vi "Looper.vi"(8 "error in (no error)":errorcluster, 11 "RSA in":refnum<class "RSA.lvclass">) -> (0 "error out":errorcluster, 3 "RSA out":refnum<class "RSA.lvclass">)   [LabVIEW 2012, in "RSA.lvclass"]
uses:
  RSA.lvclass
  <vilib>/Distrio/Murmex/GenericMessage/GenericMessage.lvclass
  <vilib>/Distrio/Murmex/Murmex/Murmex.lvclass
  <vilib>/Distrio/Murmex/ResetMessage/ResetMessage.lvclass
  <vilib>/Distrio/Murmex/StopMessage/StopMessage.lvclass
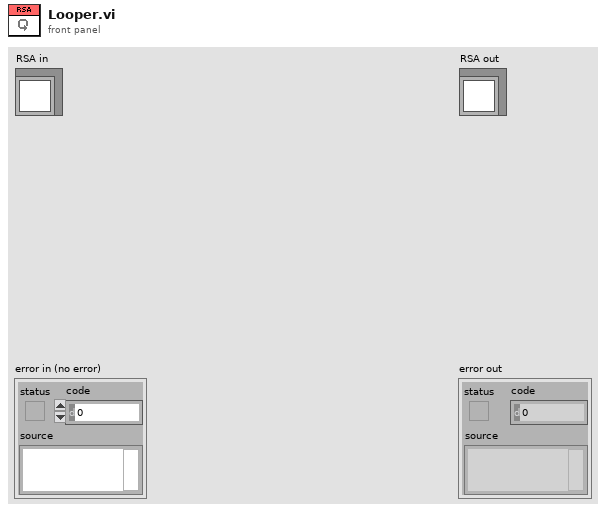
[diagram p1: front panel]
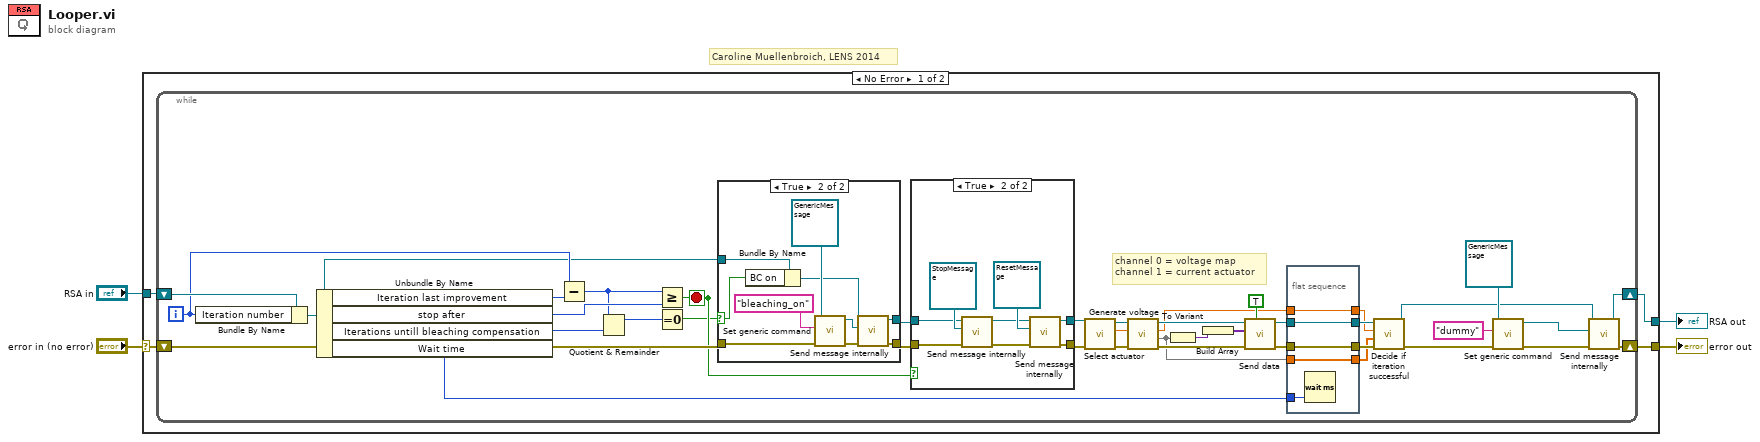
[diagram p0: block diagram]
diagram:
  # "Caroline Muellenbroich, LENS 2014"
  n1 = case shown="No Error" "error in (no error)" {
    selector: "error in (no error)" -> [w7 w77]
    tunnel: [w5 w77] -> w3
    tunnel: [w6 w76] -> w1
    tunnel: "RSA in" -> [w8 w76]
    frame No Error {
      n2 = while {
        shift-right: [w16] -> w6
        shift-left: w8 -> [w48]
        shift-right: [w15] -> w5
        shift-left: w7 -> [w44]
        i -> [w47]
        stop <- w40 stop-if-true
        # "channel 0 = voltage map\nchannel 1 = current actuator"
        n3 = Bundle By Name(cluster=w48, "Iteration number"=w47) -> (w45:refnum<class "RSA.lvclass">)
        n4 = Unbundle By Name(w45) -> ("Iteration last improvement"=w41:i32, "stop after"=w46:i32, "Iterations untill bleaching compensation"=w25:i32, "Wait time"=w27:u32)
        n5 = Subtract(x=w47, y=w41) -> (x-y=w26:i32)
        n6 = Quotient & Remainder(x=w26, y=w25) -> (x-y*floor(x/y)=w24:i32)  [unwired: 1 out]
        n7 = Greater Or Equal?(x=w26, y=w46) -> (x >= y?=w40:bool)
        n8 = Equal To 0?(x=w24) -> (x = 0?=w18:bool)
        n9 = case shown="True" w18 {
          selector: w18 -> [_ w56]
          tunnel: w45 -> [w55 w59]
          tunnel: [w55 w61] -> w42
          tunnel: w44 -> [w54 w62]
          tunnel: [w54 w60] -> w43
          frame False {
          }
          frame True {
            n10 = Bundle By Name(cluster=w59, "BC on"=w56) -> (w58:refnum<class "RSA.lvclass">)
            n11 = call <vilib>:"Set generic command.vi"("error in (no error)"=w62, "generic command"="bleaching_on", "GenericMessage in"=refnum<class "GenericMessage.lvclass"> refnum ("Murmex.lvlib:GenericMessage")) -> ("error out"=w64:errorcluster, "GenericMessage out"=w57:refnum<class "GenericMessage.lvclass">)  [unwired: 7 in]
            n12 = call <vilib>:"Send message internally.vi"("error in (no error)"=w64, "Message"=w57, "Murmex in"=w58) -> ("error out"=w60:errorcluster, "Murmex out"=w61:refnum<class "RSA.lvclass">)  [unwired: 7 in]
          }
        }
        n13 = case shown="True" w40 {
          tunnel: w43 -> [w66 w72]
          tunnel: w42 -> [w67 w69]
          tunnel: [w67 w75] -> w17
          tunnel: [w66 w74] -> w39
          frame False {
          }
          frame True {
            n14 = call <vilib>:"Send message internally.vi"("error in (no error)"=w72, "Message"=refnum<class "StopMessage.lvclass"> refnum ("Murmex.lvlib:StopMessage"), "Murmex in"=w69) -> ("error out"=w71:errorcluster, "Murmex out"=w68:refnum<class "RSA.lvclass">)  [unwired: 7 in]
            n15 = call <vilib>:"Send message internally.vi"("error in (no error)"=w71, "Message"=refnum<class "ResetMessage.lvclass"> refnum ("Message in"), "Murmex in"=w68) -> ("error out"=w74:errorcluster, "Murmex out"=w75:refnum<class "RSA.lvclass">)  [unwired: 7 in]
          }
        }
        n16 = call-dynamic "Select actuator.vi"("error in (no error)"=w39, "RSA in"=w17) -> ("error out"=w22:errorcluster, "actuatorout"=w21:dbl, "RSA out"=w23:refnum<class "RSA.lvclass">)  [unwired: 7 in]
        n17 = call "Generate voltage.vi"("error in (no error)"=w22, "Actuatorin"=w21, "RSA in"=w23) -> ("error out"=w36:errorcluster, 1:w29, "actuator out"=w20:dbl, "RSA out"=w37:refnum<class "RSA.lvclass">)  [unwired: 5 in]
        n18 = To Variant(anything=w29) -> (Variant=w38:variant)
        n19 = Build Array(w38) -> (w35:variant[])
        n20 = call <vilib>:"Send data.vi"("is finalised data? (T)"=TRUE, "error in (no error)"=w36, "data (channels array)"=w35, "Murmex in"=w37) -> ("error out"=w33:errorcluster, "Murmex out"=w31:refnum<class "RSA.lvclass">)  [unwired: 6 in]
        n21 = flat-sequence {
          tunnel: w33 -> [w53]
          tunnel: [w53] -> w32
          tunnel: w31 -> [w52]
          tunnel: [w52] -> w30
          tunnel: w29 -> [w51]
          tunnel: [w51] -> w28
          tunnel: w27 -> [w50]
          tunnel: w20 -> [w49]
          tunnel: [w49] -> w19
          frame #0 {
            n22 = Wait (ms)(milliseconds to wait=w50) -> ()  [unwired: 1 out]
          }
        }
        n23 = call-dynamic "Decide if iteration successful.vi"("error in (no error)"=w32, "current plus 1 in"=w28, "actuator in"=w19, "RSA in"=w30) -> ("error out"=w12:errorcluster, "RSA out"=w9:refnum<class "RSA.lvclass">)  [unwired: 6 in]
        n24 = call <vilib>:"Set generic command.vi"("error in (no error)"=w12, "generic command"="dummy", "GenericMessage in"=refnum<class "GenericMessage.lvclass"> refnum ("Murmex.lvlib:GenericMessage")) -> ("error out"=w11:errorcluster, "GenericMessage out"=w10:refnum<class "GenericMessage.lvclass">)  [unwired: 7 in]
        n25 = call <vilib>:"Send message internally.vi"("error in (no error)"=w11, "Message"=w10, "Murmex in"=w9) -> ("error out"=w15:errorcluster, "Murmex out"=w16:refnum<class "RSA.lvclass">)  [unwired: 7 in]
      }
    }
    frame Error {
    }
  }
  "error out" <- w3
  "RSA out" <- w1
